vi "ROI entry screen-LBox shortcut actions.vi"(8 "error in (no error)":errorcluster, 11 "ROI LBox Actions":T5=enum."Copy_current_plane") -> (0 "error out":errorcluster, 3 "ROI Info":T1 {"ROIs Info []"."FOV" min=1.0 max=10.0 step=1.0; "ROIs Info []"."Frame Size" min=1.0 max=10.0 step=1.0; "ROIs Info []"."Laser Power" min=1.0 max=10.0 step=0.10000000149011612; "ROIs Info []"."Rel. Resolution" min=1.0 max=10.0 step=1.0; "ROIs Info []"."POI Dwell time" min=1.0 max=10.0 step=0.10000000149011612; "ROIs Info []"."Zoom" min=1.0 max=10.0 step=0.10000000149011612; "Last Image Display Event info"."Tool" items=["None", "Selection Tool", "Point Tool", "Line Tool", "Rectangle Tool", "Oval Tool", "Polygon Tool", "ClosedFreehandTool", "Annulus Tool", "Rotated Rectangle Tool", "Zoom Tool", "Pan Tool", "Polyline Tool", "Freehand Tool"]; "Last Image Display Event info"."Type" items=["No Event"=0, "Click Event"=1, "Draw Event"=2, "Size Event"=4, "Scroll Event"=5, "Double Click Event"=8]})   [LabVIEW 2020]
uses:
  Typedefs/ROI Lbox actions.ctl
  Subpanel Windows/SubVIs/Typedefs/ROI Entry screen VI interface 1.ctl
  Typedefs/Last Image Display Event info.ctl
  Typedefs/ROI spec.ctl
  Typedefs/ROI ID Enum.ctl
  Typedefs/ROI management FG states.ctl
  Globals/gl_ROI Entry UI globals.vi
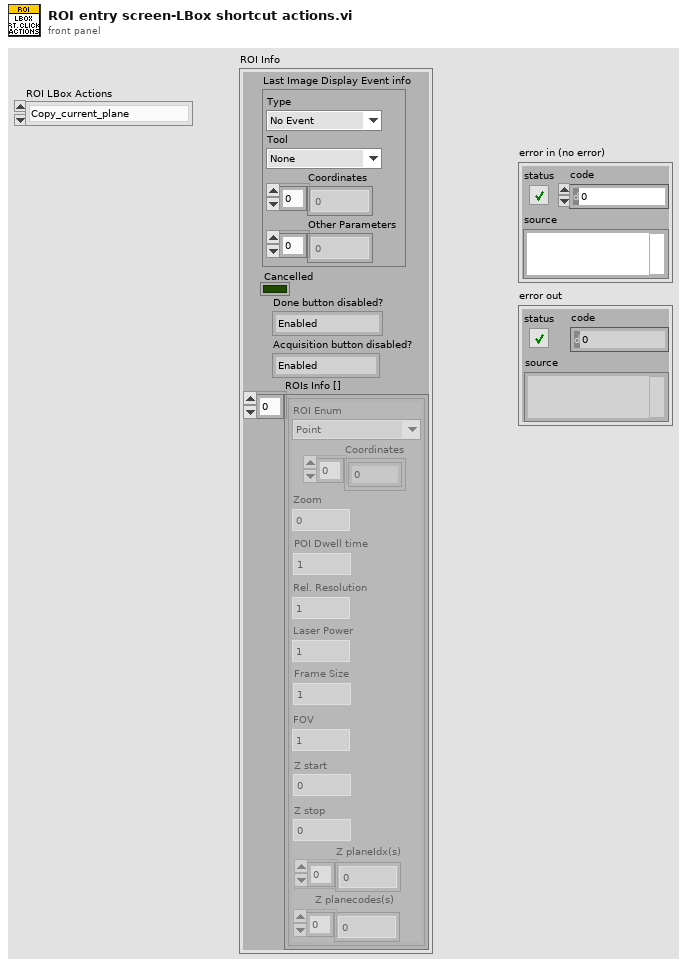
[diagram p1: front panel]
types:
  T1 = typedef "ROI Entry screen VI interface 1.ctl" = cluster{"Last Image Display Event info":T2, "ROIs Info []":T3[], "Cancelled":bool, "Done button disabled?":enum8{"Enabled", "Disabled", "Disabled and Grayed Out"}, "Acquisition button disabled?":enum8{"Enabled", "Disabled", "Disabled and Grayed Out"}}
  T2 = typedef "Last Image Display Event info.ctl" = cluster{"Type":i32, "Tool":i32, "Coordinates":i32[], "Other Parameters":sgl[]}
  T3 = typedef "ROI spec.ctl" = cluster{"ROI Enum":T4, "Coordinates":i32[], "Zoom":dbl, "POI Dwell time":dbl, "Rel. Resolution":dbl, "Laser Power":dbl, "Frame Size":dbl, "FOV":dbl, "Z start":dbl, "Z stop":dbl, "Z planeIdx(s)":i32[], "Z planecodes(s)":u8[]}
  T4 = typedef "ROI ID Enum.ctl" = enum16{"Point", "MiniScan", "Comp. MiniScan", "Rectangle", "Comp. volume", "Arb. plane point", "None"}
  T5 = typedef "ROI Lbox actions.ctl" = enum16{"Idle", "Insert", "Insert_current_plane", "Copy", "Copy_current_plane", "Replicate", "Replicate_current_plane"}
  T6 = typedef "ROI entry screen ctrl refs cluster.ctl" = cluster{"Done button":refnum<vi>, "Imaging button":refnum<vi>, "Acquisition button":refnum<vi>, "Scan dwell time per pixel (us)":refnum<vi>, "# of planes":refnum<vi>, "Zoom Ctrl":refnum<vi>, "Equal size":refnum<vi>, "Channel":refnum<vi>, "Image Display":refnum<vi>, "Z-Plane Selector":refnum<vi>, "Number of lines left":refnum<vi>, "Z-stack folder path":refnum<vi>, "POI Density":refnum<vi>, "Arb Plane Entry":refnum<vi>, "Whole Plane":refnum<vi>, "Line Mode":refnum<vi>, "Clear Last":refnum<vi>, "Clear All":refnum<vi>, "Delete Lines":refnum<vi>, "Trial Length (sec)":refnum<vi>, "Palette Type":refnum<vi>, "Intensity slider":refnum<vi>, "# POI":refnum<vi>, "Max Z Proj":refnum<vi>, "Zplane ind":refnum<vi>, "Wavelength (nm)":refnum<vi>, "Number of Trials":refnum<vi>, "Funct stim.trig.enable":refnum<vi>, "Funct stim.trig.delay (s)":refnum<vi>, "Line Mode":refnum<vi>, "Step size (µm)":refnum<vi>, "ROI move mode":refnum<vi>, "Cool-down time (s)":refnum<vi>, "Enable cool-down time":refnum<vi>, "Motor Z ind. (um)":refnum<vi>, "AOL Z ind. (um)":refnum<vi>, "Load Reference Image":refnum<vi>, "Rel.  Res.":refnum<vi>, "ROI LIST":refnum<vi>, "Show All":refnum<vi>, "ROI Type":refnum<vi>, "Start Plane":refnum<vi>, "Stop Plane":refnum<vi>, "Offset ROI":refnum<vi>, "Tab Control":refnum<vi>, "Laser Power(%)":refnum<vi>, "Cycle rate":refnum<vi>, "FOV (Ind.)":refnum<vi>, "Frame Size (Ind.)":refnum<vi>, "Resolution (Ind.)":refnum<vi>, "Pixel Density (Ind)":refnum<vi>, "Laser Power (Ind.)":refnum<vi>, "Dwell Time (Ind.)":refnum<vi>, "Adj MC":refnum<vi>}
  T7 = typedef "ROI management FG states.ctl" = enum16{"Read", "Write", "Write-from dataset", "Clear Last", "Clear All", "Delete ROI", "Update ROIs time", "Reload last ROI set", "Modify ROI Parameters", "Offset all ROI", "Offset visible ROI", "Modify Dwell Time", "Modify Laser Power"}
  T8 = typedef "ROI parameters data type.ctl" = cluster{"ROI index":dbl, "ROI ID":dbl, "ROI Time (ns)":dbl, "Pixels in ROI":dbl, "X start":dbl, "Y start":dbl, "Z start":dbl, "X stop":dbl, "Y stop":dbl, "Z stop":dbl, "Angle (deg)":dbl, "Composite ID":dbl, "Number of lines":dbl, "Frame Size":dbl, "Zoom":dbl, "Laser Power (%)":dbl, "ROI group ID":dbl, "Resolution":dbl, "Dwell Time per pixel":dbl, "Pixels per miniscan":dbl, "Original FOV (um)":dbl, "Apparent Frame Size":dbl, "Z Plane Idx":i32[], "Z Plane codes":i32[]}
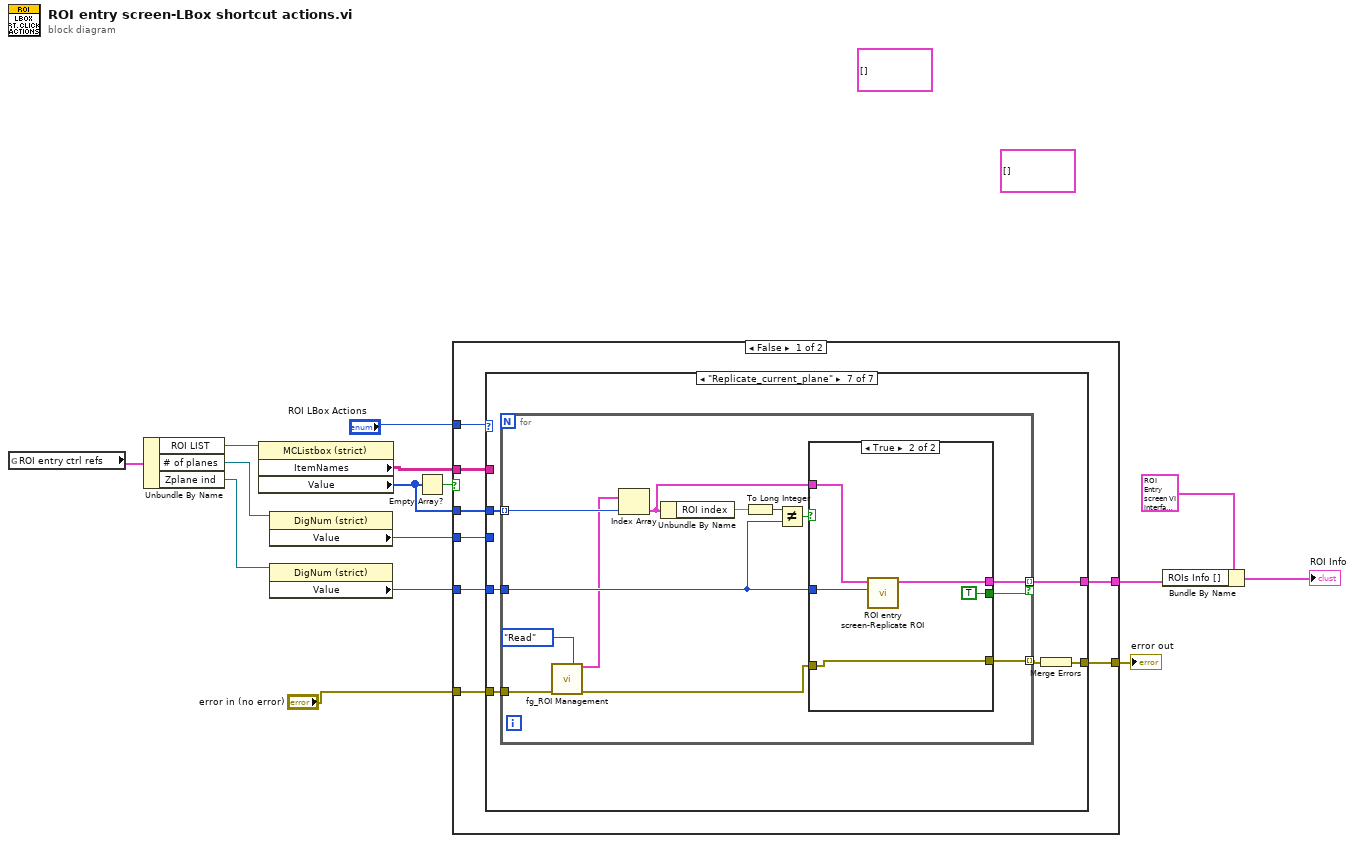
[diagram p0: block diagram]
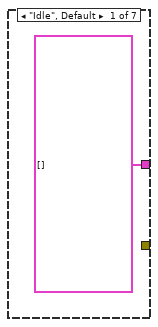
[diagram p2: hidden frame]
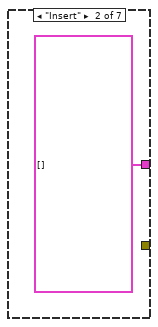
[diagram p3: hidden frame]
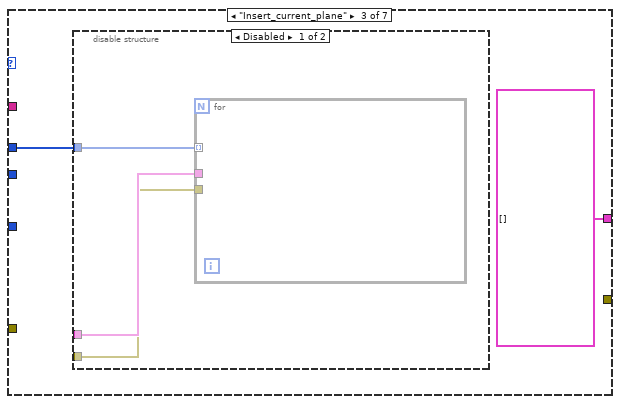
[diagram p4: hidden frame]
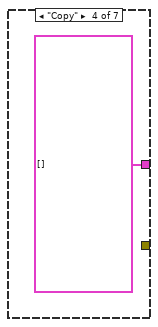
[diagram p6: hidden frame]
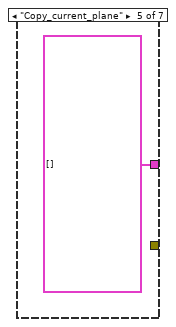
[diagram p7: hidden frame]
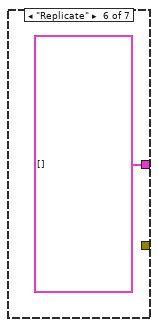
[diagram p8: hidden frame]
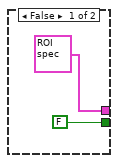
[diagram p9: hidden frame]
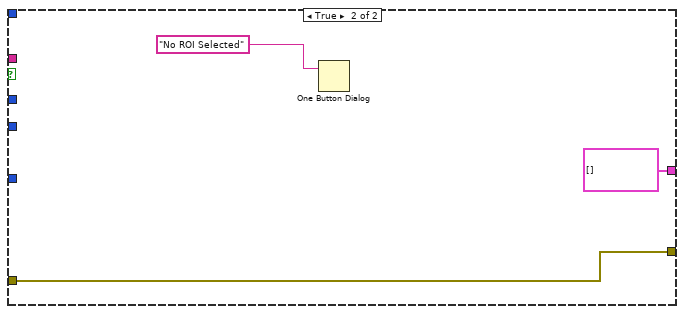
[diagram p10: hidden frame]
diagram:
  (unwired) T1[] [] ("Input cluster")
  (unwired) T1[] [] ("Input cluster")
  n1 = global read "gl_ROI Entry UI globals.vi" "ROI entry ctrl refs"() -> (w15:T6)
  n2 = Unbundle By Name(w15) -> ("ROI LIST"=w14:refnum<vi>, "# of planes"=w9:refnum<vi>, "Zplane ind"=w7:refnum<vi>)
  n3 = property class="MCListbox (strict)"(reference=w14) -> ("ItemNames"=w13:string[][], "Value"=w10:i32[])  [unwired: 1 in, 2 out]
  n4 = property class="DigNum (strict)"(reference=w9) -> ("Value"=w8:i32)  [unwired: 1 in, 2 out]
  n5 = property class="DigNum (strict)"(reference=w7) -> ("Value"=w6:i32)  [unwired: 1 in, 2 out]
  n6 = Empty Array?(array=w10) -> (empty?=w12:bool)
  n7 = case shown="False" w12 {
    tunnel: w13 -> [w22 _]
    tunnel: "ROI LBox Actions" -> [w23 _]
    tunnel: w10 -> [w21 _]
    tunnel: w8 -> [w20 _]
    tunnel: w6 -> [w19 _]
    tunnel: [w18 w60] -> w5
    tunnel: "error in (no error)" -> [w17 w60]
    tunnel: [w16 T3[] []] -> w2
    frame False {
      n8 = case shown="\"Replicate_current_plane\"" w23 {
        tunnel: w22 -> [_ _ _ _ _ _ _]
        tunnel: w21 -> [_ _ w27 _ _ _ w38]
        tunnel: w20 -> [_ _ _ _ _ _ _]
        tunnel: w19 -> [_ _ _ _ _ _ w39]
        tunnel: [_ _ _ _ _ _ w36] -> w18
        tunnel: w17 -> [_ _ _ _ _ _ w35]
        tunnel: [T3[] [] T3[] [] T3[] [] T3[] [] T3[] [] T3[] [] w34] -> w16
        frame "Idle", Default {
        }
        frame "Insert" {
        }
        frame "Insert_current_plane" {
          n9 = disable-structure shown="Disabled" {
            disable-tunnel: _ -> [w30 _]
            disable-tunnel: _ -> [w29 _]
            disable-tunnel: w27 -> [w28 _]
            frame Disabled {
              n10 = for {
                tunnel: w30 -> [_]
                tunnel: w29 -> [_]
                tunnel: w28 -> [_] mode=indexing
              }
            }
            frame Enabled {
            }
          }
        }
        frame "Copy" {
        }
        frame "Copy_current_plane" {
        }
        frame "Replicate" {
        }
        frame "Replicate_current_plane" {
          n11 = for {
            tunnel: w39 -> [w47]
            tunnel: w38 -> [w52] mode=indexing
            tunnel: [w46] -> w37 mode=indexing
            tunnel: w35 -> [w44]
            tunnel: [w41] -> w34 mode=indexing if=w40
            n12 = call "fg_ROI Management.vi"("Function"=ROI_management_FG_states."Read", "error in (no error)"=w44) -> ("ROI Setup"=w43:T8[], "error out"=w42:errorcluster)  [unwired: 7 in, 5 out]
            n13 = Index Array(array=w43, index=w52) -> (element=w48:T8)
            n14 = Unbundle By Name(w48) -> ("ROI index"=w51:dbl)
            n15 = To Long Integer(number=w51) -> (32bit integer=w50:i32)
            n16 = Not Equal?(x=w50, y=w47) -> (x != y?=w49:bool)
            n17 = case shown="True" w49 {
              tunnel: w48 -> [_ w59]
              tunnel: w47 -> [_ w58]
              tunnel: w42 -> [_ w57]
              tunnel: [_ w57] -> w46
              tunnel: [T3 {"ROI Enum"=enum."Point", "Coordinates"=[], "Zoom"=1.0, "POI Dwell time"=1.0, "Rel. Resolution"=1.0, "Laser Power"=1.0, "Frame Size"=1.0, "FOV"=1.0, "Z start"=0.0, "Z stop"=0.0, "Z planeIdx(s)"=[], "Z planecodes(s)"=[]} ("ROI info") w56] -> w41
              tunnel: [FALSE TRUE] -> w40
              frame False {
              }
              frame True {
                n18 = call "ROI entry screen-Replicate ROI.vi"("New Z plane"=w58, "XYZ"=w59) -> ("ROI info"=w56:T3)  [unwired: 8 in, 1 out]
              }
            }
          }
          n19 = Merge Errors(w37) -> (w36:errorcluster)
        }
      }
    }
    frame True {
      n20 = One Button Dialog(message="No ROI Selected") -> ()  [unwired: 1 in, 1 out]
    }
  }
  "error out" <- w5
  n21 = Bundle By Name(cluster=T1 {"Last Image Display Event info"={"Type"=0, "Tool"=0, "Coordinates"=[], "Other Parameters"=[]}, "ROIs Info []"=[], "Cancelled"=FALSE, "Done button disabled?"=enum."Enabled", "Acquisition button disabled?"=enum."Enabled"} ("Input cluster"), "ROIs Info []"=w2) -> (→"ROI Info":T1)
